vi "Acquiring Image Indicator.vi"(10 "Period":i64, 11 "Current Image":path) -> (3 "Acquiring Image":bool)   [LabVIEW 2020]
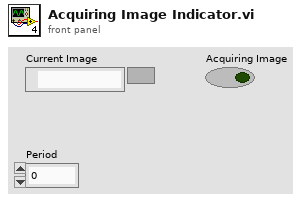
[diagram p1: front panel]
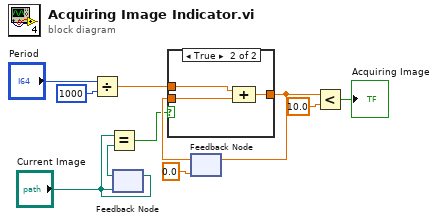
[diagram p0: block diagram]
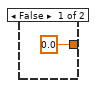
[diagram p2: hidden frame]
diagram:
  n1 = Divide(x="Period", y=i64 1000) -> (x/y=w6:dbl)
  n2 = feedback #1("Current Image") -> (w1:path)
  n3 = Equal?(x="Current Image", y=w1) -> (x = y?=w4:bool)
  n4 = feedback-in #1("Current Image") -> ()
  n5 = feedback #2(0.0) -> (w11:dbl)
  n6 = case shown="True" w4 {
    tunnel: w6 -> [_ w15]
    tunnel: [0.0 w14] -> w10
    tunnel: w11 -> [_ w13]
    frame False {
    }
    frame True {
      n7 = Compound Arithmetic op=ADD(w15, w13) -> (w14:dbl)
    }
  }
  n8 = feedback-in #2(w10) -> ()
  n9 = Less?(x=w10, y=10.0) -> (x < y?=→"Acquiring Image":bool)
